vi "lv NET获取周月日.vi"() -> ()   [LabVIEW 2018]
panel:
  out "GetWeekOfYear":i32
  in  "Time Stamp":timestamp
  in  "rule":i32(ring) items=["FirstDay", "FirstFullWeek", "FirstFourDayWeek"]
  in  "firstDayOfWeek":i32(ring) items=["Sunday", "Monday", "Tuesday", "Wednesday", "Thursday", "Friday", "Saturday"]
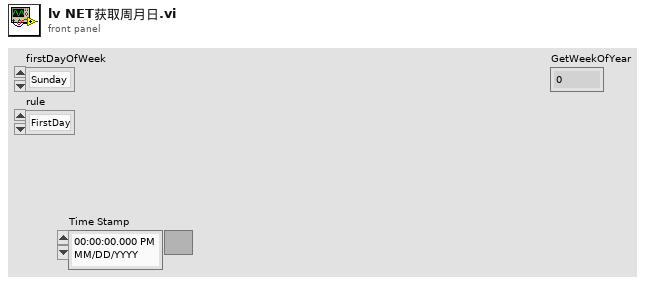
[diagram p1: front panel]
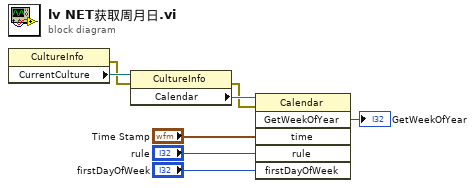
[diagram p0: block diagram]
diagram:
  n1 = property class="CultureInfo"() -> (error out=w2:errorcluster, "CurrentCulture"=w4:refnum<k24>)  [unwired: 2 in, 1 out]
  n2 = property class="CultureInfo"(reference=w4, error in=w2) -> (error out=w1:errorcluster, "Calendar"=w3:refnum<k24>)  [unwired: 1 out]
  n3 = invoke class="Calendar" method="GetWeekOfYear"(reference=w3, error in=w1, "time"="Time Stamp", "rule"="rule", "firstDayOfWeek"="firstDayOfWeek") -> ("GetWeekOfYear"=→"GetWeekOfYear":i32)  [unwired: 1 in, 5 out]
